vi "Mix Vectors.vi"(1 "inputVectors":cluster{dbl, dbl}[](array[cluster]), 4 "feildCentric":bool, 5 "x value":dbl=0.1, 6 "y value":dbl=0.1) -> (2 "finalVectors":dbl[](array[numeric]))   [LabVIEW 2018]
uses:
  swerveData.vi
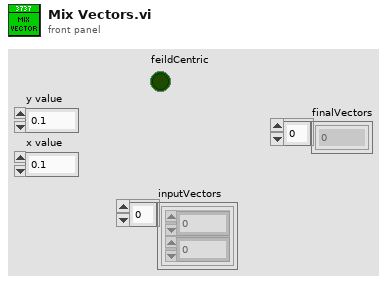
[diagram p1: front panel]
types:
  T1 = cluster{"[0]":dbl, "[1]":dbl, "[2]":dbl, "[3]":dbl, "[4]":dbl, "[5]":dbl, "[6]":dbl, "[7]":dbl, "[8]":dbl}
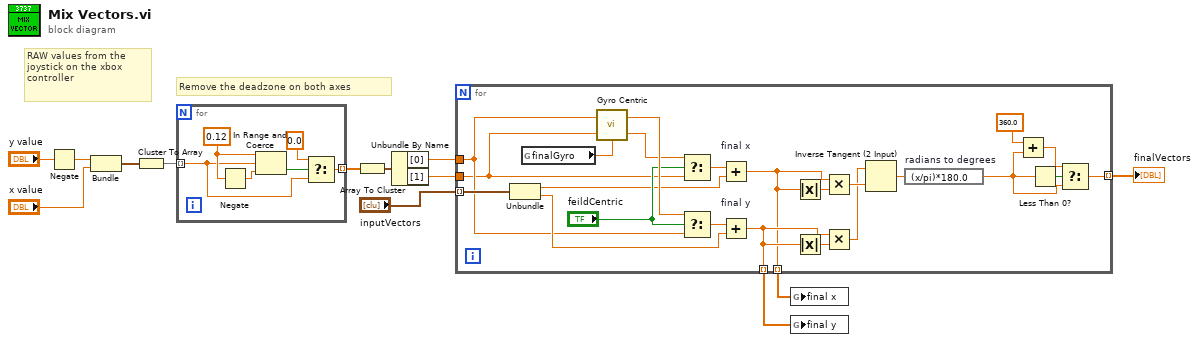
[diagram p0: block diagram]
diagram:
  # "Remove the deadzone on both axes"
  # "RAW values from the joystick on the xbox controller"
  n1 = Negate(x="y value") -> (-x=w10:dbl)
  n2 = Bundle(w10, "x value"="x value") -> (w11:cluster{dbl, "x value":dbl})  [unwired: 1 in]
  n3 = Cluster To Array(cluster=w11) -> (array=w3:dbl[])
  n4 = for {
    tunnel: w3 -> [w15] mode=indexing
    tunnel: [w14] -> w2 mode=indexing
    w17 = 0.12 ("lower limit")
    n5 = Negate(x=w17) -> (-x=w18:dbl)
    n6 = In Range and Coerce(upper limit=w17, x=w15, lower limit=w18) -> (In Range?=w19:bool)  [unwired: 1 out]
    n7 = Select(t=0.0, s=w19, f=w15) -> (s? t:f=w14:dbl)
  }
  n8 = Array To Cluster(array=w2) -> (cluster=w4:T1)
  n9 = Unbundle By Name(w4) -> ("[0]"=w5:dbl, "[1]"=w6:dbl)
  n10 = for {
    tunnel: "inputVectors" -> [w32] mode=indexing
    tunnel: [w31] -> w1 mode=indexing
    tunnel: w5 -> [w23]
    tunnel: w6 -> [w22]
    tunnel: [w20] -> w8 mode=indexing
    tunnel: [w21] -> w9 mode=indexing
    n11 = Unbundle(w32) -> (w24:dbl, w25:dbl)
    n12 = global read "swerveData.vi" "finalGyro"() -> (w33:dbl)
    n13 = call "Gyro Centric.vi"("X"=w22, "Gyro"=w33, "Y"=w23) -> ("X'"=w34:dbl, "Y'"=w42:dbl)  [unwired: 1 in]
    n14 = Select(t=w34, s="feildCentric", f=w22) -> (s? t:f=w27:dbl)
    n15 = Select(t=w42, s="feildCentric", f=w23) -> (s? t:f=w26:dbl)
    n16 = Add "final x"(x=w27, y=w24) -> (x+y=w20:dbl)
    n17 = Add "final y"(x=w26, y=w25) -> (x+y=w21:dbl)
    n18 = Absolute Value(x=w20) -> (abs(x)=w40:dbl)
    n19 = Absolute Value(x=w21) -> (abs(x)=w41:dbl)
    n20 = Multiply(x=w20, y=w40) -> (x*y=w29:dbl)
    n21 = Multiply(x=w21, y=w41) -> (x*y=w28:dbl)
    n22 = Inverse Tangent (2 Input)(1:w29, 2:w28) -> (0:w36:dbl)
    n23 = expression code="(x/pi)*180.0" "radians to degrees"(w36) -> (w35:dbl)
    n24 = Add(x=360.0, y=w35) -> (x+y=w38:dbl)
    n25 = Less Than 0?(x=w35) -> (x < 0?=w39:bool)
    n26 = Select(t=w38, s=w39, f=w35) -> (s? t:f=w31:dbl)
  }
  "finalVectors" <- w1
  n27 = global write "swerveData.vi" "final x"(w8) -> ()
  n28 = global write "swerveData.vi" "final y"(w9) -> ()
